vi "Reorder Node Children.vi"(8 "error in":errorcluster, 9 "new index":i32, 10 "current index":i32, 11 "parent section in":T1=18446744073709551615 format="%.0x") -> (0 "error out":errorcluster)   [LabVIEW 2020, in "Routing and Faulting System Explorer.lvlib"]
uses:
  Routing and Faulting System Explorer.lvlib
  <vilib>/NI VeriStand/Custom Device API/Custom Device Item Ref.ctl
  NationalInstruments.VeriStand.SystemDefinitionAPI
  NationalInstruments.VeriStand.SystemStorage
  <vilib>/NI VeriStand/Custom Device API/Custom Device API.lvlib
panel:
  out "parent section out":T1=18446744073709551615 format="%.0x"
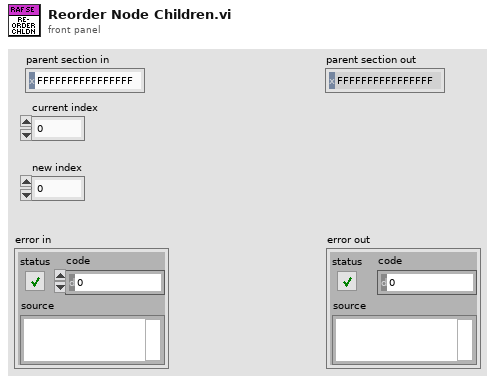
[diagram p1: front panel]
types:
  T1 = typedef "Custom Device API.lvlib/Custom Device Item Ref.ctl" = u64
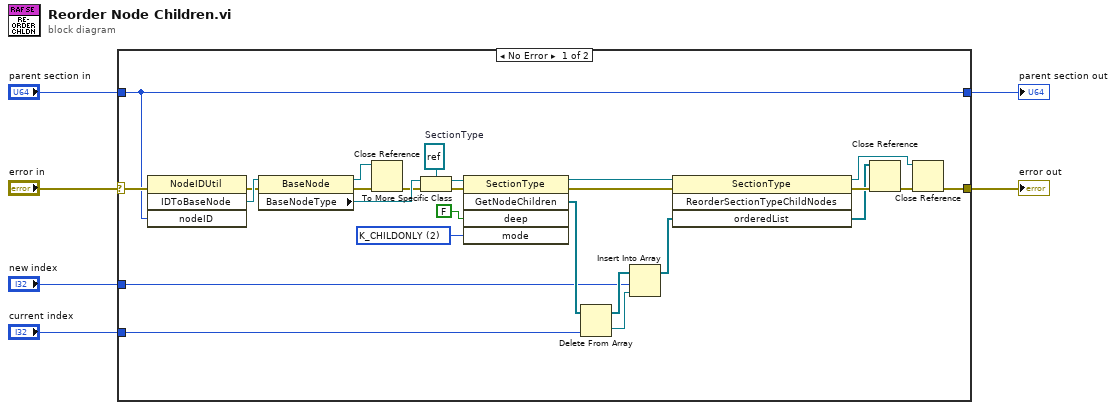
[diagram p0: block diagram]
diagram:
  n1 = case shown="No Error" "error in" {
    selector: "error in" -> [w9 w34]
    tunnel: "current index" -> [w25 _]
    tunnel: "new index" -> [w22 _]
    tunnel: [w8 w34] -> w3
    tunnel: "parent section in" -> [w7 w33]
    tunnel: [w7 w33] -> w1
    frame No Error {
      w27 = 2 items=["K_BFS", "K_DFS", "K_CHILDONLY", "K_UP"] ("mode")
      w30 = refnum<k24> refnum  # SectionType
      n2 = invoke class="NodeIDUtil" method="IDToBaseNode"(error in=w9, "nodeID"=w7) -> (error out=w18:errorcluster, "IDToBaseNode"=w32:refnum<k24>)  [unwired: 2 in, 2 out]
      n3 = property class="BaseNode"(reference=w32, error in=w18) -> (reference out=w16:refnum<k24>, error out=w17:errorcluster, "BaseNodeType"=w31:refnum<k24>)
      n4 = Close Reference(reference=w16, error in (no error)=w17) -> (error out=w15:errorcluster)
      n5 = To More Specific Class(target class=w30, reference=w31, error in=w15) -> (specific class reference=w29:refnum<k24>, error out=w14:errorcluster)
      n6 = invoke class="SectionType" method="GetNodeChildren"(reference=w29, error in=w14, "deep"=FALSE, "mode"=w27) -> (reference out=w13:refnum<k24>, error out=w10:errorcluster, "GetNodeChildren"=w26:refnum<k24>[])  [unwired: 1 in, 2 out]
      n7 = Delete From Array(array=w26, index=w25) -> (deleted portion=w23:refnum<k24>, array with subset deleted=w24:refnum<k24>[])  [unwired: 1 in]
      n8 = Insert Into Array(array=w24, index=w22, new element=w23) -> (w21:refnum<k24>[])
      n9 = invoke class="SectionType" method="ReorderSectionTypeChildNodes"(reference=w13, error in=w10, "orderedList"=w21) -> (reference out=w12:refnum<k24>, error out=w20:errorcluster, "orderedList"=w19:refnum<k24>[])  [unwired: 1 in, 1 out]
      n10 = Close Reference(reference=w19, error in (no error)=w20) -> (error out=w11:errorcluster)
      n11 = Close Reference(reference=w12, error in (no error)=w11) -> (error out=w8:errorcluster)
    }
    frame Error {
    }
  }
  "error out" <- w3
  "parent section out" <- w1
